vi "Resonance 1.vi"() -> ()   [LabVIEW 2021]
panel:
  out "pressure DMM reading":dbl
  out "?":dbl(graph)
  out "Pressure":dbl
  in  "Output File Name":path=path "test.lvm" caption="Filename"
  out "?":cluster{"Y":dbl[], "Y":dbl[]}[](graph)
  out "Current Frequency =":dbl
  out "Excitation =":dbl
  out "Progress":u8(slide) scale=0.0..100.0
  in  "number of steps":dbl
  in  "stop frequency (Hz)":dbl
  in  "start frequency (Hz)":dbl
  out "?":dbl(graph)
  out "?":dbl(graph)
  out "Temperature":string
  in  "Scan Speed":T1(ring)
  out "Resonance Amplitude":string
  # "Hz"
  # "mV"
  # "C"
  # "torr"
  # "microV"
  # "V"
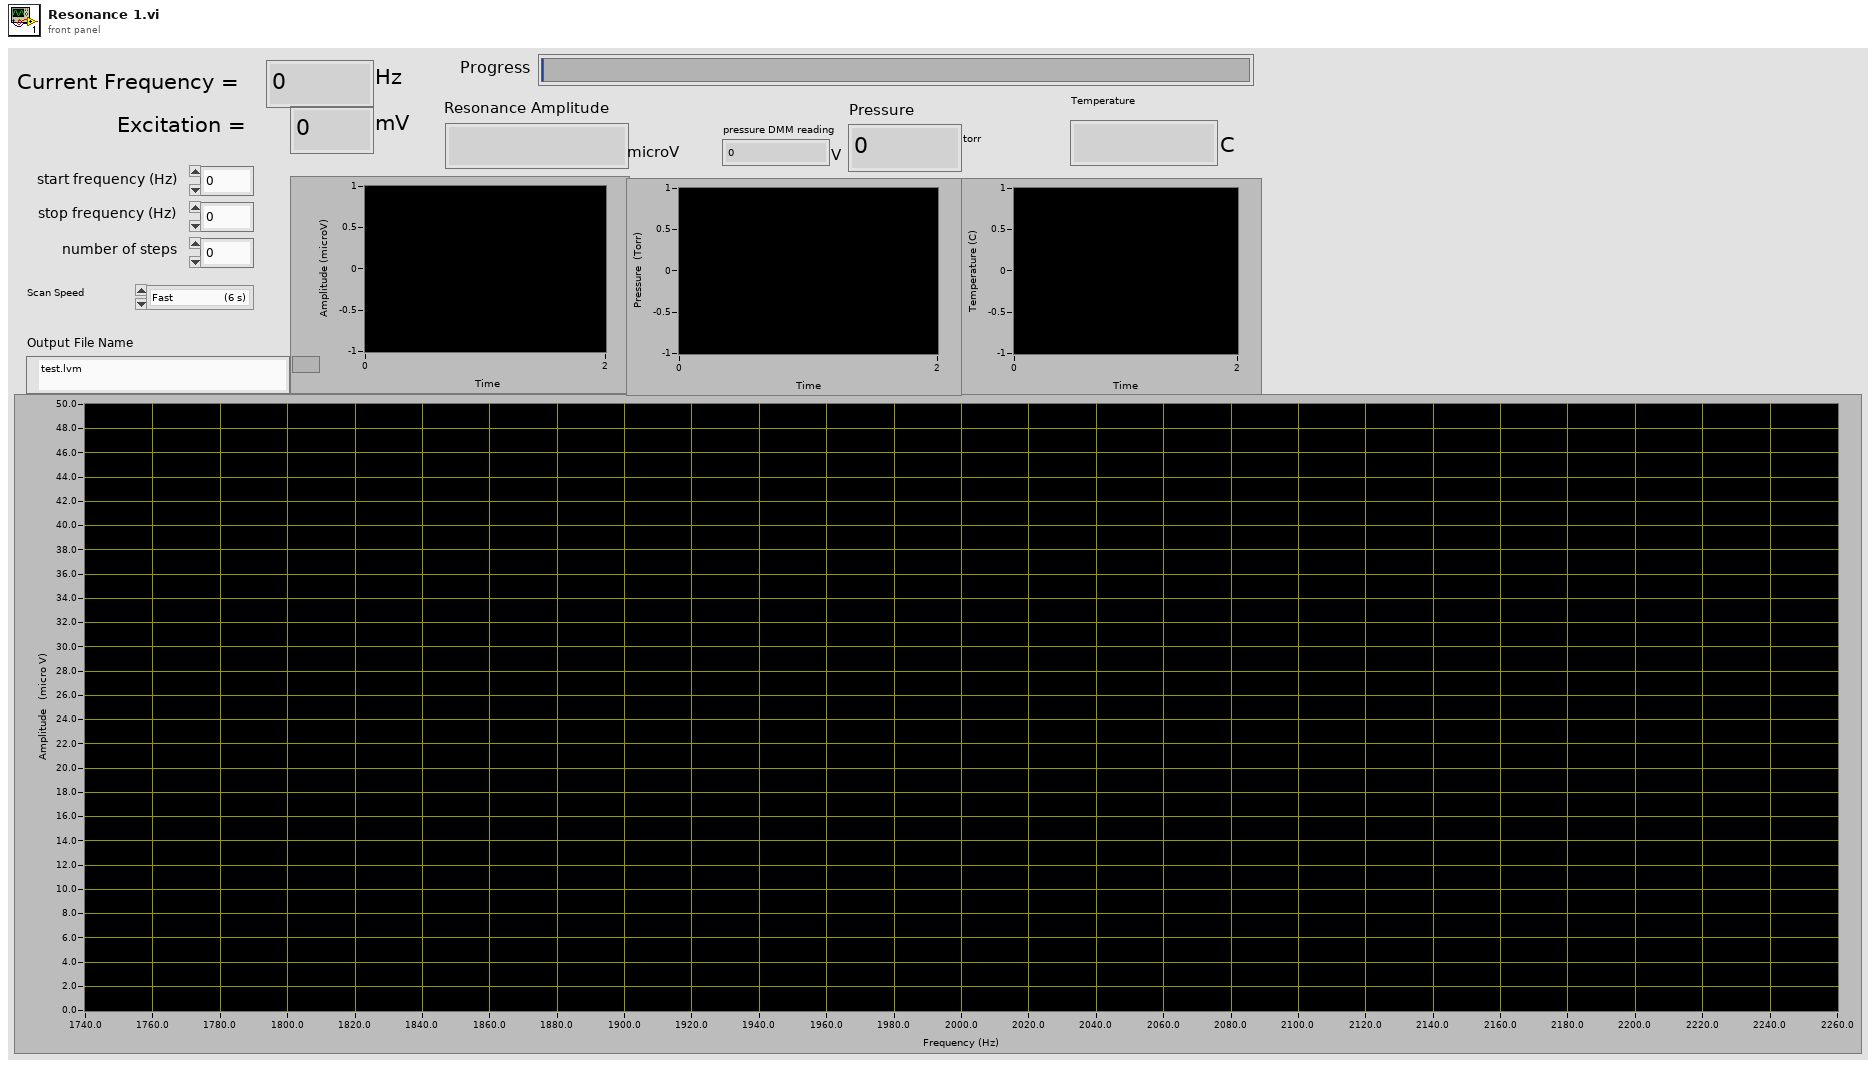
[diagram p1: front panel]
types:
  T1 = enum16{"Fast                 (6 s)", "Slow              (15 s)", "Very Slow  (1 min)"}
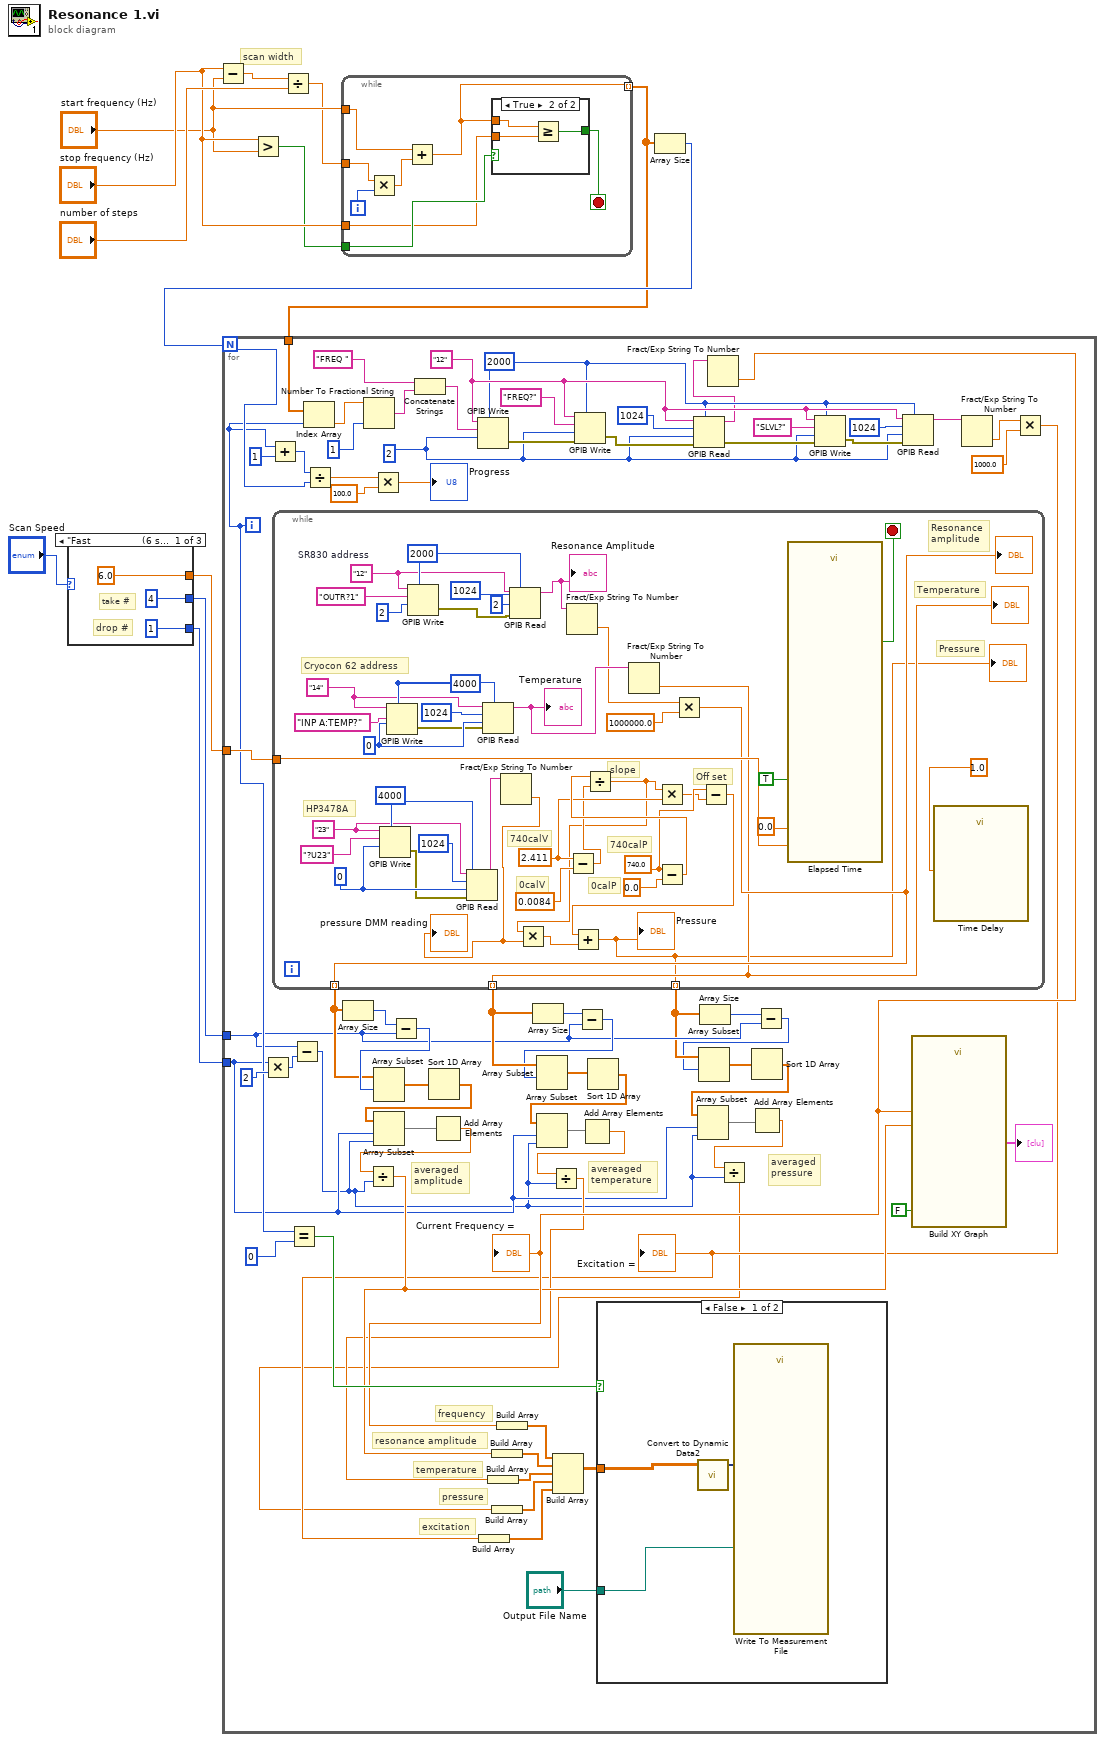
[diagram p0: block diagram]
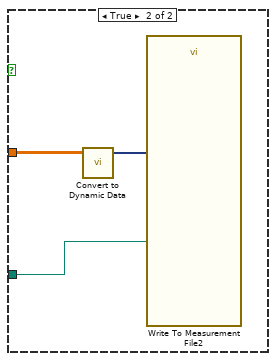
[diagram p2: hidden frame]
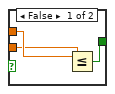
[diagram p3: hidden frame]
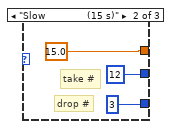
[diagram p4: hidden frame]
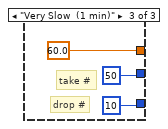
[diagram p5: hidden frame]
diagram:
  # "scan width"
  n1 = case shown="\"Fast                 (6 s)\", Default" "Scan Speed" {
    tunnel: [6.0 15.0 60.0] -> w11
    tunnel: [1 3 10] -> w1
    tunnel: [4 12 50] -> w2
    frame "Fast                 (6 s)", Default {
      # "take #"
      # "drop #"
    }
    frame "Slow              (15 s)" {
      # "take #"
      # "drop #"
    }
    frame "Very Slow  (1 min)" {
      # "take #"
      # "drop #"
    }
  }
  n2 = Subtract(x="stop frequency (Hz)", y="start frequency (Hz)") -> (x-y=w10:dbl)
  n3 = Greater?(x="stop frequency (Hz)", y="start frequency (Hz)") -> (0:w6:bool)
  n4 = Divide(x=w10, y="number of steps") -> (x/y=w5:dbl)
  n5 = while {
    tunnel: "start frequency (Hz)" -> [w29]
    tunnel: w5 -> [w23]
    tunnel: "stop frequency (Hz)" -> [w25]
    tunnel: w6 -> [w26]
    tunnel: [w22] -> w3 mode=indexing
    i -> [w28]
    stop <- w24 stop-if-true
    n6 = Multiply(x=w23, y=w28) -> (x*y=w27:dbl)
    n7 = Add(x=w29, y=w27) -> (x+y=w22:dbl)
    n8 = case shown="True" w26 {
      tunnel: w22 -> [w32 w35]
      tunnel: w25 -> [w31 w34]
      tunnel: [w30 w33] -> w24
      frame False {
        n9 = Less Or Equal?(x=w32, y=w31) -> (x <= y?=w30:bool)
      }
      frame True {
        n10 = Greater Or Equal?(x=w35, y=w34) -> (x >= y?=w33:bool)
      }
    }
  }
  n11 = Array Size(array=w3) -> (size(s)=w4:i32)
  n12 = for {
    N: w4 -> [w93]
    tunnel: w11 -> [w106]
    tunnel: w3 -> [w105]
    tunnel: w2 -> [w46]
    tunnel: w1 -> [w41]
    i -> [w60]
    w84 = "12" ("address string")
    w86 = i16 2 ("mode (0)")
    w83 = 2000 ("timeout ms (488.2 global)")
    # "excitation"
    # "pressure"
    # "averaged\npressure"
    # "temperature"
    # "resonance amplitude"
    # "frequency"
    # "avereaged\ntemperature"
    # "averaged\namplitude"
    n13 = Multiply(x=w41, y=2) -> (x*y=w77:i32)
    n14 = Add(x=w60, y=1) -> (x+y=w94:i32)
    n15 = while {
      tunnel: w106 -> [w144]
      tunnel: [w133] -> w73 mode=indexing
      tunnel: [w132] -> w68 mode=indexing
      tunnel: [w114] -> w45 mode=indexing
      stop <- w135 stop-if-true
      w120 = 740.0
      w121 = 2.411
      w127 = i16 0 ("mode (0)")
      w130 = 4000 ("timeout ms (488.2 global)")
      w129 = "23" ("address string")
      w141 = i16 0 ("mode (0)")
      w142 = "14" ("address string")
      w143 = 4000 ("timeout ms (488.2 global)")
      w146 = 2000 ("timeout ms (488.2 global)")
      w145 = "12"  # SR830 address
      # "Resonance\namplitude"
      # "Temperature"
      # "Pressure"
      # "Off set"
      # "slope"
      # "740calP"
      # "740calV"
      # "0calP"
      # "0calV"
      # "HP3478A"
      # "Cryocon 62 address"
      n16 = GPIB Write(0:w129, 1:"?U23" ("data"), 2:w127, 4:w130) -> (6:w126:errorcluster)  [unwired: 1 in, 1 out]
      n17 = GPIB Write(0:w142, 1:"INP A:TEMP?" ("data"), 2:w141, 4:w143) -> (6:w140:errorcluster)  [unwired: 1 in, 1 out]
      n18 = GPIB Write(0:w145, 1:"OUTR?1" ("data"), 2:i16 2 ("mode (0)"), 4:w146) -> (6:w152:errorcluster)  [unwired: 1 in, 1 out]
      n19 = GPIB Read(0:w129, 1:1024 ("byte count"), 2:w127, 3:w126, 4:w130) -> (5:w125:string)  [unwired: 2 out]
      n20 = GPIB Read(0:w142, 1:1024 ("byte count"), 2:w141, 3:w140, 4:w143) -> (5:w136:string)  [unwired: 2 out]
      "Temperature" <- w136
      n21 = Fract/Exp String To Number(string=w125) -> (number=w113:dbl)  [unwired: 3 in, 1 out]
      "pressure DMM reading" <- w113
      n22 = GPIB Read(0:w145, 1:1024 ("byte count"), 2:i16 2 ("mode (0)"), 3:w152, 4:w146) -> (5:w137:string)  [unwired: 2 out]
      "Resonance Amplitude" <- w137
      n23 = Fract/Exp String To Number(string=w137) -> (number=w134:dbl)  [unwired: 3 in, 1 out]
      n24 = Subtract(x=w121, y=0.0084) -> (x-y=w116:dbl)
      n25 = Fract/Exp String To Number(string=w136) -> (number=w132:dbl)  [unwired: 3 in, 1 out]
      "?" <- w132
      n26 = Subtract(x=w120, y=0.0) -> (x-y=w122:dbl)
      n27 = Divide(x=w122, y=w116) -> (x/y=w115:dbl)
      n28 = Multiply(x=w115, y=w113) -> (x*y=w118:dbl)
      n29 = Multiply(x=w115, y=w121) -> (x*y=w119:dbl)
      n30 = Multiply(x=w134, y=1000000.0) -> (x*y=w133:dbl)
      "?" <- w133
      n31 = Subtract(x=w120, y=w119) -> (x-y=w117:dbl)
      n32 = Add(x=w117, y=w118) -> (x+y=w114:dbl)
      "Pressure" <- w114
      "?" <- w114
      n33 = call "Elapsed Time"("Time Target (s)"=w144, "Auto Reset"=TRUE, "Set Start Time (s)"=0.0) -> ("Time has Elapsed"=w135:bool)  [unwired: 9 in, 7 out]
      n34 = call "Time Delay"("Delay Time (s)"=1.0) -> ()  [unwired: 10 in, 1 out]
    }
    n35 = Equal?(x=w60, y=0) -> (x = y?=w58:bool)
    n36 = Subtract(x=w46, y=w77) -> (x-y=w38:i32)
    n37 = Index Array(array=w105, index=w60) -> (element=w103:dbl)
    n38 = Divide(x=w94, y=w93) -> (x/y=w92:dbl)
    n39 = Array Size(array=w73) -> (size(s)=w76:i32)
    n40 = Number To Fractional String(number=w103, precision (6)=i16 1) -> (F-format string=w100:string)  [unwired: 2 in]
    n41 = Multiply(x=w92, y=100.0) -> (x*y=→"Progress":dbl)
    n42 = Subtract(x=w76, y=w46) -> (x-y=w75:i32)
    n43 = Array Subset(array=w73, index=w75) -> (w74:dbl[])  [unwired: 1 in]
    n44 = Concatenate Strings("FREQ " ("string"), w100) -> (w101:string)
    n45 = Sort 1D Array(array=w74) -> (sorted array=w72:dbl[])
    n46 = Array Subset(array=w72, index=w41, length=w38) -> (w70:dbl[])
    n47 = Add Array Elements(numeric array=w70) -> (sum=w71:dbl)
    n48 = Divide(x=w71, y=w38) -> (x/y=w53:dbl)
    n49 = GPIB Write(0:w84, 1:w101, 2:w86, 4:w83) -> (6:w96:errorcluster)  [unwired: 1 in, 1 out]
    n50 = Build Array(w53) -> (w52:dbl[])
    n51 = Array Size(array=w68) -> (size(s)=w69:i32)
    n52 = GPIB Write(0:w84, 1:"FREQ?" ("data"), 2:w86, 3:w96, 4:w83) -> (6:w97:errorcluster)  [unwired: 1 out]
    n53 = Subtract(x=w69, y=w46) -> (x-y=w67:i32)
    n54 = Array Subset(array=w68, index=w67) -> (w66:dbl[])  [unwired: 1 in]
    n55 = Sort 1D Array(array=w66) -> (sorted array=w65:dbl[])
    n56 = Array Subset(array=w65, index=w41, length=w38) -> (w64:dbl[])
    n57 = Add Array Elements(numeric array=w64) -> (sum=w63:dbl)
    n58 = Divide(x=w63, y=w38) -> (x/y=w51:dbl)
    n59 = Build Array(w51) -> (w50:dbl[])
    n60 = GPIB Read(0:w84, 1:1024 ("byte count"), 2:w86, 3:w97, 4:w83) -> (5:w79:string, 7:w88:errorcluster)  [unwired: 1 out]
    n61 = Array Size(array=w45) -> (size(s)=w47:i32)
    n62 = Fract/Exp String To Number(string=w79) -> (number=w55:dbl)  [unwired: 3 in, 1 out]
    "Current Frequency =" <- w55
    n63 = Build Array(w55) -> (w54:dbl[])
    n64 = Subtract(x=w47, y=w46) -> (x-y=w44:i32)
    n65 = Array Subset(array=w45, index=w44) -> (w43:dbl[])  [unwired: 1 in]
    n66 = Sort 1D Array(array=w43) -> (sorted array=w42:dbl[])
    n67 = Array Subset(array=w42, index=w41, length=w38) -> (w40:dbl[])
    n68 = Add Array Elements(numeric array=w40) -> (sum=w39:dbl)
    n69 = Divide(x=w39, y=w38) -> (x/y=w36:dbl)
    n70 = Build Array(w36) -> (w37:dbl[])
    n71 = GPIB Write(0:w84, 1:"SLVL?" ("data"), 2:w86, 3:w88, 4:w83) -> (6:w87:errorcluster)  [unwired: 1 out]
    n72 = GPIB Read(0:w84, 1:1024 ("byte count"), 2:w86, 3:w87, 4:w83) -> (5:w82:string)  [unwired: 2 out]
    n73 = call "Build XY Graph"("Reset"=FALSE, "Y Input"=w53, "X Input"=w55) -> ("XY Graph"=→"?":cluster{"X":dbl[], "Y":dbl[]}[])  [unwired: 7 in, 1 out]
    n74 = Fract/Exp String To Number(string=w82) -> (number=w81:dbl)  [unwired: 3 in, 1 out]
    n75 = Multiply(x=w81, y=1000.0) -> (x*y=w49:dbl)
    "Excitation =" <- w49
    n76 = Build Array(w49) -> (w48:dbl[])
    n77 = Build Array(w54, w52, w50, w37, w48) -> (w56:dbl[][])
    n78 = case shown="False" w58 {
      tunnel: "Output File Name" -> [w107 w112]
      tunnel: w56 -> [w109 w111]
      frame False {
        n79 = call "Convert to Dynamic Data2"("2D Array"=w109) -> ("Dynamic Data Type"=w108:dynamicdata)  [unwired: 3 in]
        n80 = call "Write To Measurement File"("Signals"=w108, "Filename"=w107) -> ()  [unwired: 15 in, 3 out]
      }
      frame True {
        n81 = call "Convert to Dynamic Data"("2D Array"=w111) -> ("Dynamic Data Type"=w110:dynamicdata)  [unwired: 3 in]
        n82 = call "Write To Measurement File2"("Signals"=w110, "Filename"=w112) -> ()  [unwired: 15 in, 3 out]
      }
    }
  }
